vi "Add Connections to State.vi"(8 "error in (no error)":errorcluster, 10 "Connection List":T1[](array[typedef]), 11 "Routing State in":T2) -> (0 "error out":errorcluster, 1 "a connection exists":bool, 3 "Routing State out":T2)   [LabVIEW 2017, in "Switch Scripting.lvlib"]
uses:
  Switch Scripting.lvlib
  Routing State.ctl
  Connection.ctl
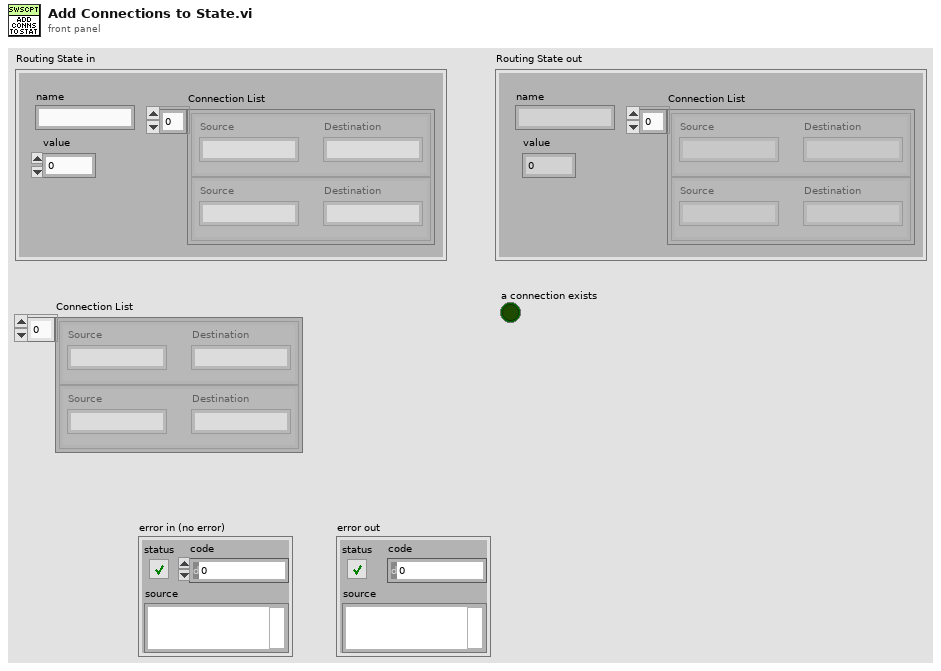
[diagram p1: front panel]
types:
  T1 = typedef "Switch Scripting.lvlib/Connection.ctl" = cluster{"Source":string, "Destination":string}
  T2 = typedef "Switch Scripting.lvlib/Routing State.ctl" = cluster{"name":string, "value":i32, "Connection List":T1[]}
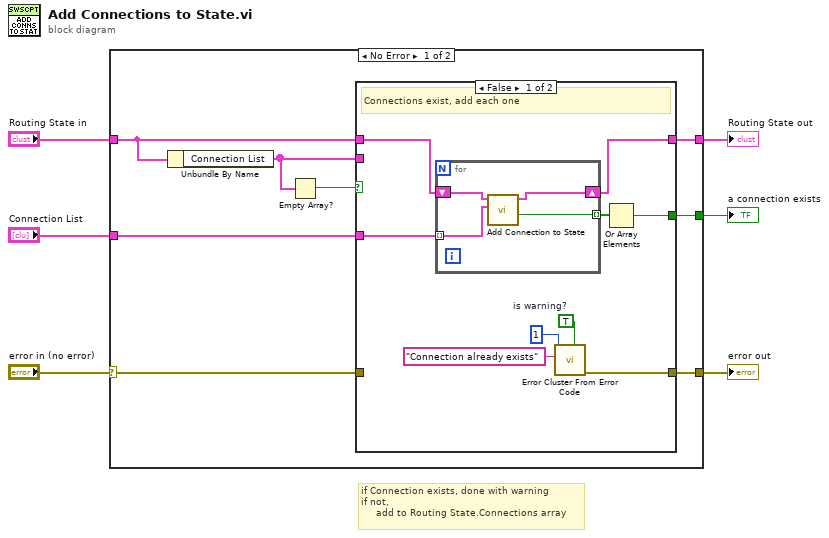
[diagram p0: block diagram]
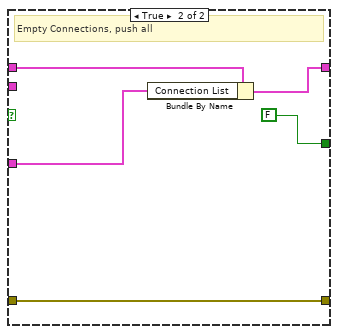
[diagram p2: hidden frame]
diagram:
  # "if Connection exists, done with warning\nif not, \n     add to Routing State.Connections array"
  n1 = case shown="No Error" "error in (no error)" {
    selector: "error in (no error)" -> [w14 w34]
    tunnel: [w13 w34] -> w6
    tunnel: [w9 w33] -> w5
    tunnel: "Routing State in" -> [w10 w33]
    tunnel: "Connection List" -> [w11 _]
    tunnel: [w12 _] -> w1
    frame No Error {
      n2 = Unbundle By Name(w10) -> ("Connection List"=w8:T1[])
      n3 = Empty Array?(array=w8) -> (empty?=w7:bool)
      n4 = case shown="False" w7 {
        tunnel: w14 -> [_ w32]
        tunnel: [w21 w32] -> w13
        tunnel: [w17 FALSE] -> w12
        tunnel: w8 -> [_ _]
        tunnel: w11 -> [w19 w28]
        tunnel: w10 -> [w16 w30]
        tunnel: [w15 w29] -> w9
        frame False {
          w22 = TRUE  # is warning?
          # "Connections exist, add each one"
          n5 = for {
            shift-right: [w26] -> w15
            shift-left: w16 -> [w27]
            tunnel: w19 -> [w25] mode=indexing
            tunnel: [w24] -> w18 mode=indexing
            n6 = call "Add Connection to State.vi"("Connection"=w25, "Routing State in"=w27) -> ("already exists"=w24:bool, "Routing State out"=w26:T2)  [unwired: 7 in, 1 out]
          }
          n7 = call <vilib>:"Error Cluster From Error Code.vi"("is warning? (False)"=w22, "error message (\"\")"="Connection already exists" ("error message (\"\")"), "error code (0)"=1) -> ("error out"=w21:errorcluster)  [unwired: 6 in]
          n8 = Or Array Elements(Boolean array=w18) -> (logical OR=w17:bool)
        }
        frame True {
          # "Empty Connections, push all"
          n9 = Bundle By Name(cluster=w30, "Connection List"=w28) -> (w29:T2)
        }
      }
    }
    frame Error {
    }
  }
  "error out" <- w6
  "Routing State out" <- w5
  "a connection exists" <- w1
